vi "Lift&Hang.vi"(8 "error in (no error)":errorcluster, 10 "status":dbl, 11 "refnum name":string="My Motor RefNum") -> (0 "error out":errorcluster)   [LabVIEW 2016]
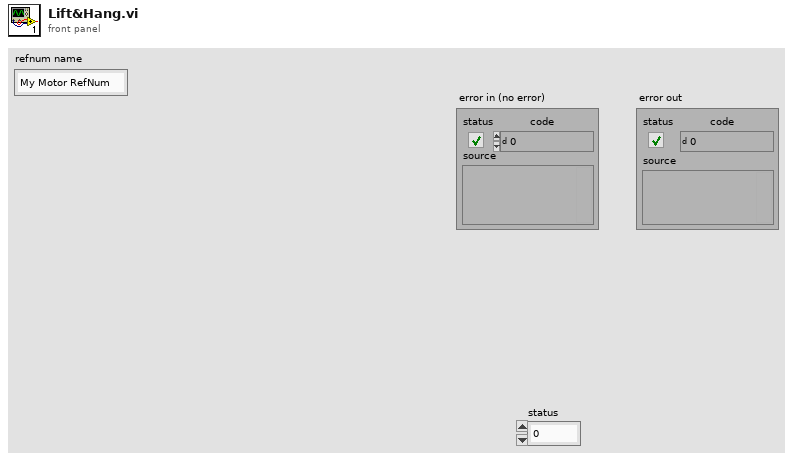
[diagram p1: front panel]
types:
  T1 = typedef "WPI_MotorControlDeviceRef.ctl" = cluster{"DeviceStatus":errorcluster, "Type":T2, "PWM":cluster{"PWM Channel":T3, "DeadBand":T4}, "CAN":cluster{"Device Number":u8, "SetOutput VI Ref":variant, "GetOutput VI Ref":variant, "Enable VI Ref":variant, "Disable VI Ref":variant, "Data":variant}, "Invert":bool}
  T2 = typedef "WPI_MotorControlType.ctl" = enum16{"PWM", "CAN"}
  T3 = typedef "FPGA_DIOPWMChannel.ctl" = enum8{"PWM 0", "PWM 1", "PWM 2", "PWM 3", "PWM 4", "PWM 5", "PWM 6", "PWM 7", "PWM 8", "PWM 9", "PWM MXP 0", "PWM MXP 1", "PWM MXP 2", "PWM MXP 3", "PWM MXP 4", "PWM MXP 5", "PWM MXP 6", "PWM MXP 7", "PWM MXP 8", "PWM MXP 9", "Invalid"}
  T4 = typedef "WPI_PWMDeadband.ctl" = cluster{"Name":string, "maxPositivePwm":i32, "minPositivePwm":i32, "centerPwm":i32, "maxNegativePwm":i32, "minNegativePwm":i32, "angularRange":u16}
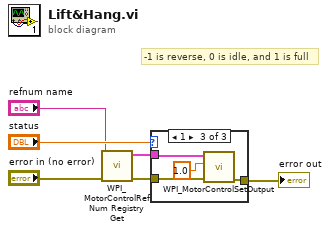
[diagram p0: block diagram]
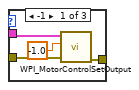
[diagram p2: hidden frame]
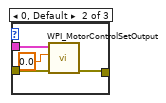
[diagram p3: hidden frame]
diagram:
  # "-1 is reverse, 0 is idle, and 1 is full"
  n1 = call <vilib>:"WPI_MotorControlRefNum Registry Get.vi"("error in (no error)"="error in (no error)", "refnum name"="refnum name") -> ("error out"=w3:errorcluster, "MotorControlDevRef"=w5:T1)  [unwired: 8 in]
  n2 = case shown="1" "status" {
    tunnel: w5 -> [w9 w14 w17]
    tunnel: w3 -> [w8 w11 w16]
    tunnel: [w7 w12 w15] -> w2
    frame -1 {
      n3 = call <vilib>:"WPI_MotorControlSetOutput.vi"("error in (no error)"=w8, "Output"=-1.0, "MotorControlDevRef"=w9) -> ("error out"=w7:errorcluster)  [unwired: 6 in, 2 out]
    }
    frame 0, Default {
      n4 = call <vilib>:"WPI_MotorControlSetOutput.vi"("error in (no error)"=w11, "Output"=0.0, "MotorControlDevRef"=w14) -> ("error out"=w12:errorcluster)  [unwired: 6 in, 2 out]
    }
    frame 1 {
      n5 = call <vilib>:"WPI_MotorControlSetOutput.vi"("error in (no error)"=w16, "Output"=1.0, "MotorControlDevRef"=w17) -> ("error out"=w15:errorcluster)  [unwired: 6 in, 2 out]
    }
  }
  "error out" <- w2
